vi "Store Ctl Refs.vi"(4 "Data":refnum<vi>, 5 "UI Refs in":T1, 6 "Status":refnum<vi>, 7 "Stop":refnum<vi>, 9 "Exit":refnum<vi>, 10 "Settings":refnum<vi>, 11 "Start":refnum<vi>) -> (1 "Disable":refnum<vi>[](array[refnum]), 2 "UI Refs out":T1, 3 "Enable":refnum<vi>[](array[refnum]))   [LabVIEW 2025]
uses:
  controls/UI Data.ctl
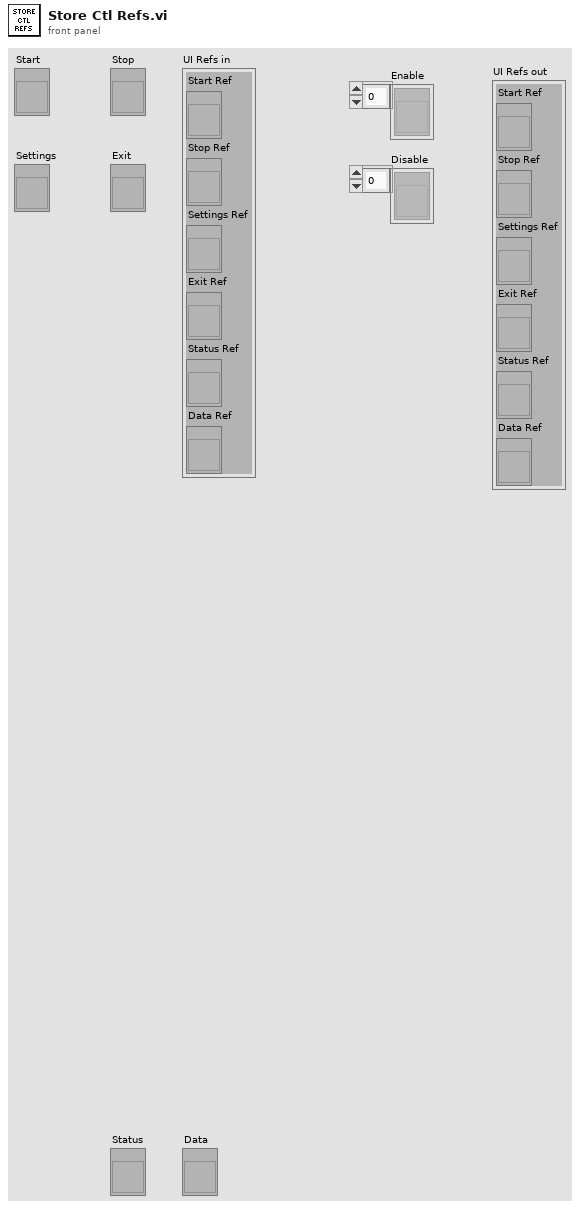
[diagram p1: front panel]
types:
  T1 = typedef "UI Data.ctl" = cluster{"Start Ref":refnum<vi>, "Stop Ref":refnum<vi>, "Settings Ref":refnum<vi>, "Exit Ref":refnum<vi>, "Status Ref":refnum<vi>, "Data Ref":refnum<vi>}
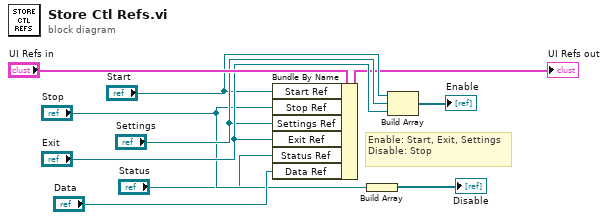
[diagram p0: block diagram]
diagram:
  # "Enable: Start, Exit, Settings\nDisable: Stop"
  n1 = Bundle By Name(cluster="UI Refs in", "Start Ref"="Start", "Stop Ref"="Stop", "Settings Ref"="Settings", "Exit Ref"="Exit", "Status Ref"="Status", "Data Ref"="Data") -> (→"UI Refs out":T1)
  n2 = Build Array("Stop") -> (→"Disable":refnum<vi>[])
  n3 = Build Array("Start", "Settings", "Exit") -> (→"Enable":refnum<vi>[])
